vi "Linear Fit.vi"   [LabVIEW 2019, in "xy_utilities.lvlib"]
doc: "Performs a linear fit using linear LS algorithm.\n\nWire data to the data input to determine the polymorphic instance to use or manually select the instance."
uses:
  xy_utilities.lvlib
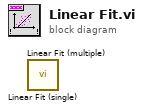
[diagram p0: block diagram]
diagram:
  n1 = call "Linear Fit (single).vi"() -> ()  [unwired: 5 in, 7 out]
  n2 = call "Linear Fit (multiple).vi"() -> ()  [unwired: 5 in, 7 out]
